vi "String Replace LabVIEW Data Types With C types.vi"(1 "C code":string) -> (0 "C code, replaced datatypes":string)   [LabVIEW 2014]
doc: "Concatenates String Array Into one String. If optional delimiter provided, it's inserted between each String Array item."
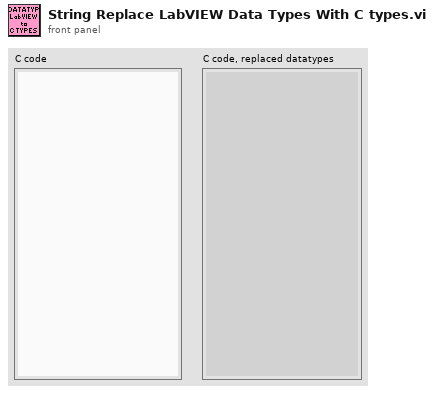
[diagram p1: front panel]
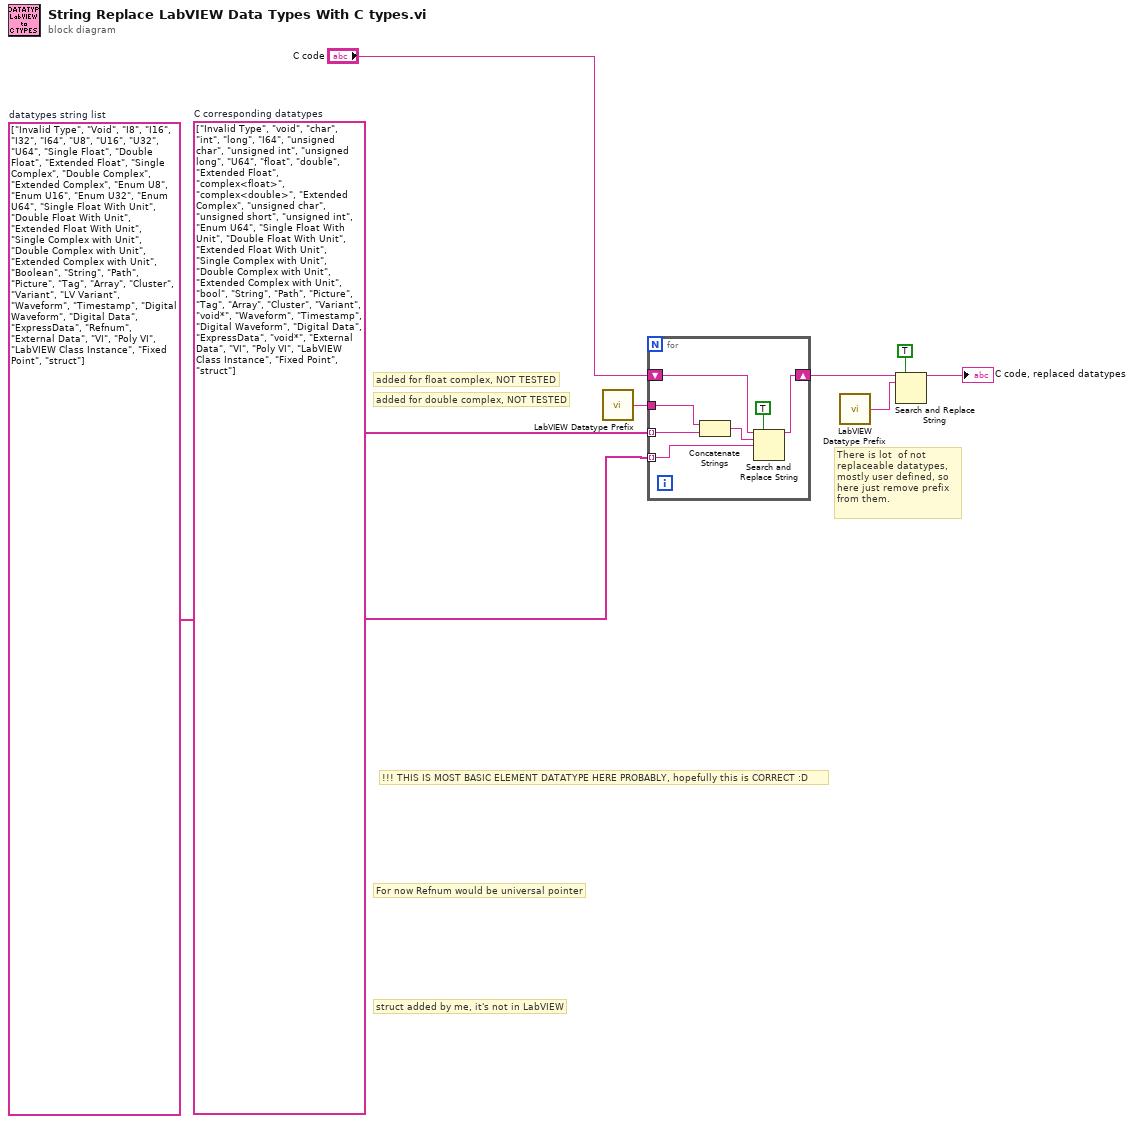
[diagram p0: block diagram]
diagram:
  w7 = string[] ["Invalid Type", "void", "char", "int", "long", "I64", "unsigned char", "unsigned int", "unsigned long", "U64", "float", "double", "Extended Float", "complex<float>", "complex<double>", "Extended Complex", "unsigned char", "unsigned short", "unsigned int", "Enum U64", "Single Float With Unit", "Double Float With Unit", "Extended Float With Unit", "Single Complex with Unit", "Double Complex with Unit", "Extended Complex with Unit", "bool", "String", "Path", "Picture", "Tag", "Array", "Cluster", "Variant", "void*", "Waveform", "Timestamp", "Digital Waveform", "Digital Data", "ExpressData", "void*", "External Data", "VI", "Poly VI", "LabVIEW Class Instance", "Fixed Point", "struct"]  # C corresponding datatypes
  w8 = string[] ["Invalid Type", "Void", "I8", "I16", "I32", "I64", "U8", "U16", "U32", "U64", "Single Float", "Double Float", "Extended Float", "Single Complex", "Double Complex", "Extended Complex", "Enum U8", "Enum U16", "Enum U32", "Enum U64", "Single Float With Unit", "Double Float With Unit", "Extended Float With Unit", "Single Complex with Unit", "Double Complex with Unit", "Extended Complex with Unit", "Boolean", "String", "Path", "Picture", "Tag", "Array", "Cluster", "Variant", "LV Variant", "Waveform", "Timestamp", "Digital Waveform", "Digital Data", "ExpressData", "Refnum", "External Data", "VI", "Poly VI", "LabVIEW Class Instance", "Fixed Point", "struct"]  # datatypes string list
  # "!!! THIS IS MOST BASIC ELEMENT DATATYPE HERE PROBABLY, hopefully this is CORRECT :D"
  # "added for double complex, NOT TESTED"
  # "added for float complex, NOT TESTED"
  # "For now Refnum would be universal pointer"
  # "There is lot  of not replaceable datatypes, mostly user defined, so here just remove prefix from them."
  # "struct added by me, it's not in LabVIEW"
  n1 = call "LabVIEW Datatype Prefix.vi"() -> ("datatype prefix"=w5:string)
  n2 = for {
    tunnel: w8 -> [w14] mode=indexing
    tunnel: w7 -> [w13] mode=indexing
    shift-right: [w11] -> w2
    shift-left: "C code" -> [w15]
    tunnel: w5 -> [w9]
    n3 = Concatenate Strings(w9, w14) -> (w10:string)
    n4 = Search and Replace String(replace all?=TRUE ("replace all? (F)"), input string=w15, search string=w10, replace string=w13) -> (result string=w11:string)  [unwired: 4 in, 3 out]
  }
  n5 = call "LabVIEW Datatype Prefix.vi"() -> ("datatype prefix"=w3:string)
  n6 = Search and Replace String(replace all?=TRUE ("replace all? (F)"), input string=w2, search string=w3) -> (result string=→"C code, replaced datatypes":string)  [unwired: 5 in, 3 out]
